vi "SwerveDrive2.0.vi"() -> ()   [LabVIEW 2020]
panel:
  out "WA 4":dbl
  out "WA 3":dbl
  out "WA 2":dbl
  out "WA 1":dbl
  out "WS 4":dbl
  out "WS 3":dbl
  out "WS 2":dbl
  out "WS 1":dbl
  in  "W4 Encoder":dbl
  in  "W3 Encoder":dbl
  in  "W2 Encoder":dbl
  in  "W1 Encoder":dbl
  in  "RCW":dbl(slide) scale=-1.0..1.0
  in  "STR":dbl(slide) scale=-1.0..1.0
  in  "FWD":dbl(slide) scale=-1.0..1.0
  in  "Gyro":dbl
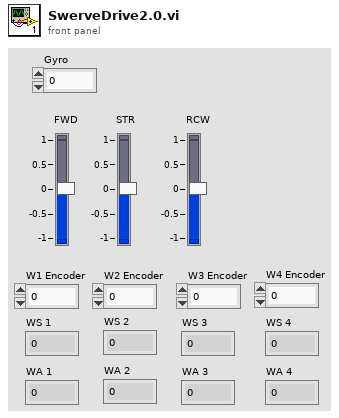
[diagram p1: front panel]
types:
  T1 = typedef "WPI_MotorControlDeviceRef.ctl" = cluster{"DeviceStatus":errorcluster, "Type":T2, "PWM":cluster{"PWM Channel":T3, "DeadBand":T4}, "CAN":cluster{"Device Number":u8, "SetOutput VI Ref":variant, "GetOutput VI Ref":variant, "Enable VI Ref":variant, "Disable VI Ref":variant, "Data":variant}, "Invert":bool, "DIO PWM":cluster{"PWM \"Enable\" Channel":T3, "DIOChannel":T5, "PWM Rate":dbl}}
  T2 = typedef "WPI_MotorControlType.ctl" = enum16{"PWM", "CAN", "DIO PWM"}
  T3 = typedef "FPGA_DIOPWMChannel.ctl" = enum8{"PWM 0", "PWM 1", "PWM 2", "PWM 3", "PWM 4", "PWM 5", "PWM 6", "PWM 7", "PWM 8", "PWM 9", "PWM MXP 0", "PWM MXP 1", "PWM MXP 2", "PWM MXP 3", "PWM MXP 4", "PWM MXP 5", "PWM MXP 6", "PWM MXP 7", "PWM MXP 8", "PWM MXP 9", "Invalid"}
  T4 = typedef "WPI_PWMDeadband.ctl" = cluster{"Name":string, "maxPositivePwm":i32, "minPositivePwm":i32, "centerPwm":i32, "maxNegativePwm":i32, "minNegativePwm":i32, "angularRange":u16}
  T5 = typedef "FPGA_DIOChannel.ctl" = enum8{"DIO 0", "DIO 1", "DIO 2", "DIO 3", "DIO 4", "DIO 5", "DIO 6", "DIO 7", "DIO 8", "DIO 9", "DIO MXP 0", "DIO MXP 1", "DIO MXP 2", "DIO MXP 3", "DIO MXP 4", "DIO MXP 5", "DIO MXP 6", "DIO MXP 7", "DIO MXP 8", "DIO MXP 9", "DIO MXP 10", "DIO MXP 11", "DIO MXP 12", "DIO MXP 13", "DIO MXP 14", "DIO MXP 15", "SPI Port CS1", "SPI Port CS2", "SPI Port CS3", "SPI Port MISO", "SPI Port MOSI", "Invalid"}
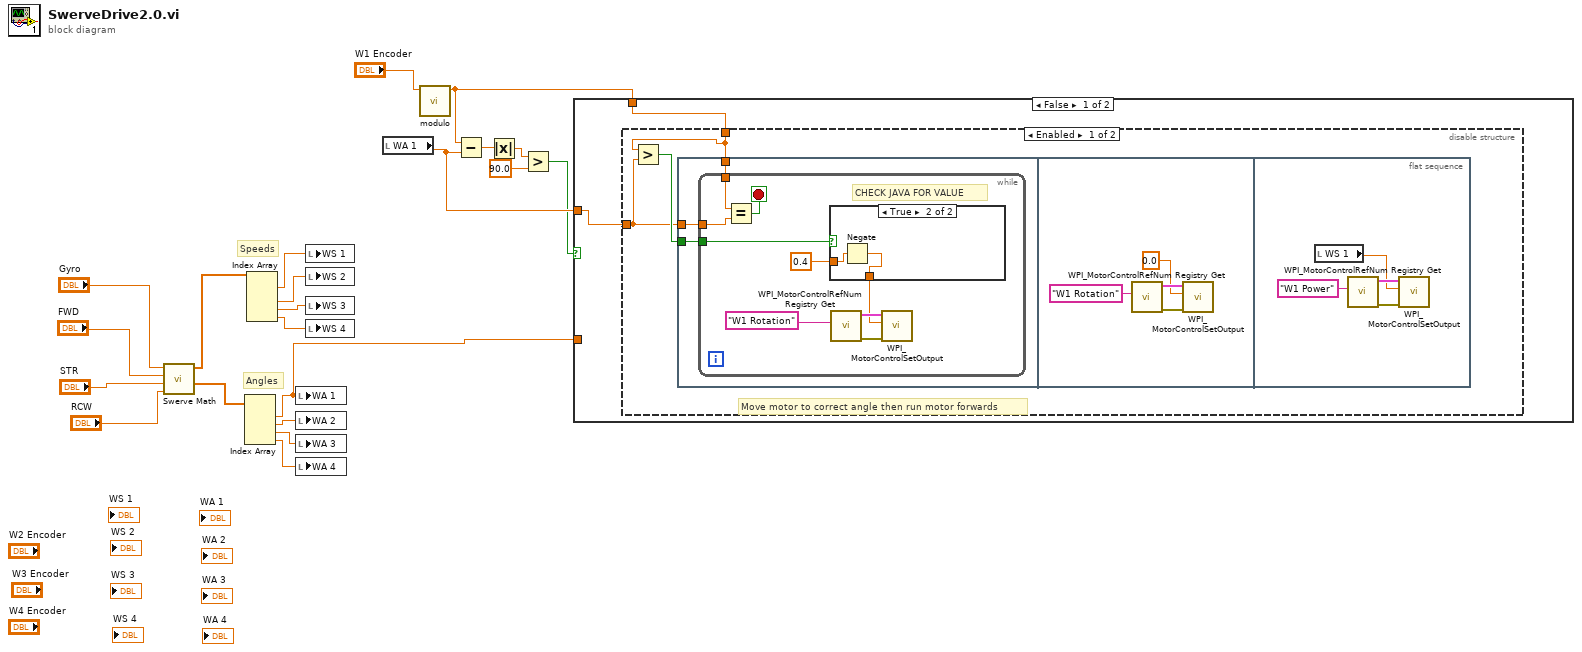
[diagram p0: block diagram]
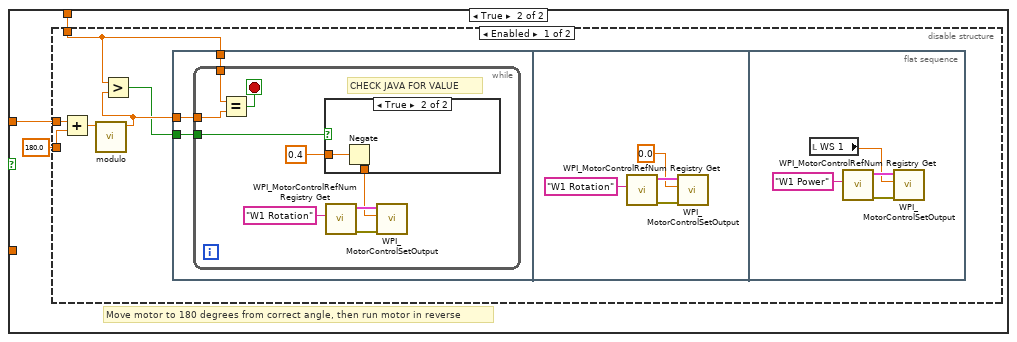
[diagram p4: hidden frame]
diagram:
  # "Angles"
  # "Speeds"
  n1 = call "Swerve Math.vi"("Gyro"="Gyro", "FWD"="FWD", "STR"="STR", "RCW"="RCW") -> ("Wheel Speeds"=w17:dbl[], "Wheel Angles"=w16:dbl[])  [unwired: 5 in]
  n2 = Index Array(array=w16) -> (element #1=w1:dbl, element #2=w14:dbl, element #3=w15:dbl, element #4=w13:dbl)  [unwired: 4 in]
  n3 = Index Array(array=w17) -> (element #1=w9:dbl, element #2=w10:dbl, element #3=w12:dbl, element #4=w11:dbl)  [unwired: 4 in]
  n4 = local write "WA 1"(w1) -> ()
  n5 = local write "WA 2"(w14) -> ()
  n6 = local write "WA 3"(w15) -> ()
  n7 = local write "WA 4"(w13) -> ()
  n8 = local write "WS 1"(w9) -> ()
  n9 = local write "WS 2"(w10) -> ()
  n10 = local write "WS 3"(w12) -> ()
  n11 = local write "WS 4"(w11) -> ()
  n12 = local read "WA 1"() -> (w4:dbl)
  n13 = call "modulo.vi"("X1"="W1 Encoder") -> ("Result"=w3:dbl)  [unwired: 10 in]
  n14 = Subtract(x=w3, y=w4) -> (x-y=w7:dbl)
  n15 = Absolute Value(x=w7) -> (abs(x)=w6:dbl)
  n16 = Greater?(x=w6, y=90.0) -> (0:w2:bool)
  n17 = case shown="False" w2 {
    tunnel: w4 -> [w22 w52]
    tunnel: w3 -> [w23 w50]
    tunnel: w1 -> [_ _]
    frame False {
      n18 = disable-structure shown="Enabled" {
        disable-tunnel: w23 -> [w25 _]
        disable-tunnel: w22 -> [w24 _]
        frame Enabled {
          # "Move motor to correct angle then run motor forwards"
          n19 = Greater?(x=w25, y=w24) -> (0:w26:bool)
          n20 = flat-sequence {
            tunnel: w25 -> [w29]
            tunnel: w24 -> [w28]
            tunnel: w26 -> [w27]
            frame #0 {
              n21 = while {
                tunnel: w29 -> [w37]
                tunnel: w28 -> [w36]
                tunnel: w27 -> [w35]
                stop <- w38 stop-if-true
                # "CHECK JAVA FOR VALUE"
                n22 = Equal?(x=w37, y=w36) -> (x = y?=w38:bool)
                n23 = case shown="True" w35 {
                  tunnel: 0.4 ("Output") -> [w39 w41]
                  tunnel: [w39 w40] -> w31
                  frame False {
                  }
                  frame True {
                    n24 = Negate(x=w41) -> (-x=w40:dbl)
                  }
                }
                n25 = call <vilib>:"WPI_MotorControlRefNum Registry Get.vi"("refnum name"="W1 Rotation") -> ("error out"=w34:errorcluster, "MotorControlDevRef"=w33:T1)  [unwired: 9 in]
                n26 = call <vilib>:"WPI_MotorControlSetOutput.vi"("error in (no error)"=w34, "Output"=w31, "MotorControlDevRef"=w33) -> ()  [unwired: 6 in, 3 out]
              }
            }
            frame #1 {
              n27 = call <vilib>:"WPI_MotorControlRefNum Registry Get.vi"("refnum name"="W1 Rotation") -> ("error out"=w44:errorcluster, "MotorControlDevRef"=w43:T1)  [unwired: 9 in]
              n28 = call <vilib>:"WPI_MotorControlSetOutput.vi"("error in (no error)"=w44, "Output"=0.0, "MotorControlDevRef"=w43) -> ()  [unwired: 6 in, 3 out]
            }
            frame #2 {
              n29 = local read "WS 1"() -> (w46:dbl)
              n30 = call <vilib>:"WPI_MotorControlRefNum Registry Get.vi"("refnum name"="W1 Power") -> ("error out"=w48:errorcluster, "MotorControlDevRef"=w47:T1)  [unwired: 9 in]
              n31 = call <vilib>:"WPI_MotorControlSetOutput.vi"("error in (no error)"=w48, "Output"=w46, "MotorControlDevRef"=w47) -> ()  [unwired: 6 in, 3 out]
            }
          }
        }
        frame Disabled {
        }
      }
    }
    frame True {
      # "Move motor to 180 degrees from correct angle, then run motor in reverse"
      n32 = disable-structure shown="Enabled" {
        disable-tunnel: w52 -> [w58 _]
        disable-tunnel: 180.0 ("y") -> [w57 _]
        disable-tunnel: w50 -> [w55 _]
        frame Enabled {
          n33 = Add(x=w58, y=w57) -> (x+y=w56:dbl)
          n34 = call "modulo.vi"("X1"=w56) -> ("Result"=w54:dbl)  [unwired: 10 in]
          n35 = Greater?(x=w55, y=w54) -> (0:w53:bool)
          n36 = flat-sequence {
            tunnel: w55 -> [w61]
            tunnel: w54 -> [w60]
            tunnel: w53 -> [w59]
            frame #0 {
              n37 = while {
                tunnel: w61 -> [w69]
                tunnel: w60 -> [w68]
                tunnel: w59 -> [w67]
                stop <- w70 stop-if-true
                # "CHECK JAVA FOR VALUE"
                n38 = Equal?(x=w69, y=w68) -> (x = y?=w70:bool)
                n39 = case shown="True" w67 {
                  tunnel: 0.4 ("Output") -> [w71 w73]
                  tunnel: [w71 w72] -> w62
                  frame False {
                  }
                  frame True {
                    n40 = Negate(x=w73) -> (-x=w72:dbl)
                  }
                }
                n41 = call <vilib>:"WPI_MotorControlRefNum Registry Get.vi"("refnum name"="W1 Rotation") -> ("error out"=w65:errorcluster, "MotorControlDevRef"=w64:T1)  [unwired: 9 in]
                n42 = call <vilib>:"WPI_MotorControlSetOutput.vi"("error in (no error)"=w65, "Output"=w62, "MotorControlDevRef"=w64) -> ()  [unwired: 6 in, 3 out]
              }
            }
            frame #1 {
              n43 = call <vilib>:"WPI_MotorControlRefNum Registry Get.vi"("refnum name"="W1 Rotation") -> ("error out"=w76:errorcluster, "MotorControlDevRef"=w75:T1)  [unwired: 9 in]
              n44 = call <vilib>:"WPI_MotorControlSetOutput.vi"("error in (no error)"=w76, "Output"=0.0, "MotorControlDevRef"=w75) -> ()  [unwired: 6 in, 3 out]
            }
            frame #2 {
              n45 = local read "WS 1"() -> (w78:dbl)
              n46 = call <vilib>:"WPI_MotorControlRefNum Registry Get.vi"("refnum name"="W1 Power") -> ("error out"=w80:errorcluster, "MotorControlDevRef"=w79:T1)  [unwired: 9 in]
              n47 = call <vilib>:"WPI_MotorControlSetOutput.vi"("error in (no error)"=w80, "Output"=w78, "MotorControlDevRef"=w79) -> ()  [unwired: 6 in, 3 out]
            }
          }
        }
        frame Disabled {
        }
      }
    }
  }
